vi "action_set.vi"(0 "reference":refnum<class "OSA.lvclass">, 2 "action data":T1[](array[typedef]) {"par 4" format="%.2f"; "par 3" format="%.2f"; "par 2" format="%.2f"; "par" format="%.2f"}, 5 "error in (no error)":errorcluster) -> (14 "duplicate reference":refnum<class "OSA.lvclass">, 19 "error out":errorcluster)   [LabVIEW 2010, in "OSA.lvclass"]
doc: "Set next action and place it in queue."
uses:
  OSA.lvclass
  misc_examples/action_data.ctl
  typeDef/queue_action.ctl
  OSA20X_misc.lvlib
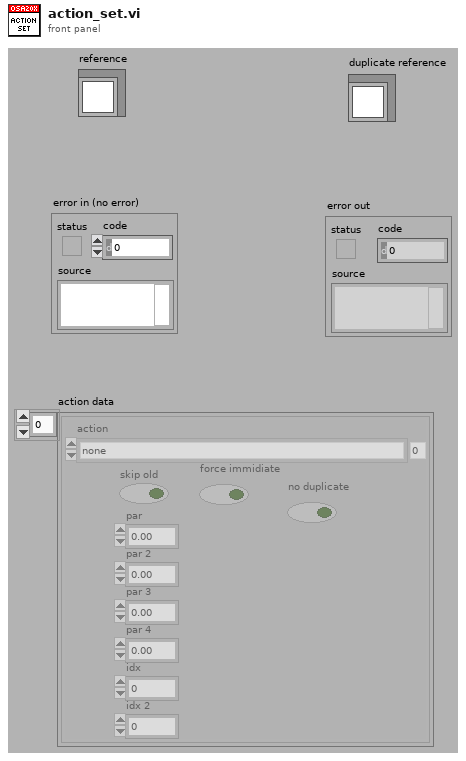
[diagram p1: front panel]
types:
  T1 = typedef "OSA.lvclass/action_data.ctl" = cluster{"action":T2, "skip old":bool, "force immidiate":bool, "par":dbl, "par 2":dbl, "par 3":dbl, "par 4":dbl, "idx":i32, "idx 2":i32, "no duplicate":bool}
  T2 = typedef "OSA.lvclass/queue_action.ctl" = enum16{"none", "stop", "GUI_plotInterferogram", "GUI_plotSpectrum", "GUI_plotInterferogramRescale", "GUI_plotSpectrumRescale", "GUI_plotInterferogramReset", "GUI_plotSpectrumReset", "GUI_plotInterferogramAutoScaleY", "GUI_plotSpectrumAutoScaleY", "GUI_plotInterferogramZoomOut", "GUI_plotSpectrumZoomOut", "GUI_plotInterferogramPane", "GUI_plotSpectrumPane", "GUI_plotInterferogramZoomMouse", "GUI_plotSpectrumZoomMouse", "ENVIRONMENT temperature", "ENVIRONMENT pressure", "MODE_resolution set", "MODE_resolution get", "MODE_sensitivity set", "MODE_sensitivity get", "MODE_PDTemperature set", "MODE_PDTemperature get", "REBOOT/RESET firmware", "ACQASYNC_acquireSingleSpectrum", "ACQASYNC_continuous start", "ACQASYNC_continuous stop\n", "ACQASYNC_get last interferogram", "ACQASYNC_get last spectrum", "ACQASYNC_get last waveNr", "ACQOPT_interferogram smoothing set", "ACQOPT_interferogram smoothing get", "ACQOPT_spectrum smoothing set", "ACQOPT_spectrum smoothing get", "ACQOPT_apodisation type set", "ACQOPT_apodisation type get", "ACQOPT_phase correction type set", "ACQOPT_phase correction type get", "ACQOPT_acqIntervall_set", "ACQOPT_acqIntervall_get", "ACQOPT_average spectrum set", "ACQOPT_average spectrum get", "ACQOPT_rolling average set", "ACQOPT_rolling average get", "ACQOPT_zero fill factor set", "ACQOPT_zero fill factor get", "ACQOPT_cycle counting set", "ACQOPT_cycle counting get", "ACQOPT_air measure option set", "ACQOPT_air measure option get", "ACQOPT_gainLevel auto get", "ACQOPT_gainLevel auto set", "ACQOPT_gainLevel get", "ACQOPT_gainLevel set", "ACQOPT_getAll", "INSTRUMENT_PROPERTY_range_WaveNr_min", "INSTRUMENT_PROPERTY_range_WaveNr_max", "INSTRUMENT_PROPERTY_reference_wavelength_cm^-1", "INSTRUMENT_PROPERTY_samplesPerRefPeriod", "INSTRUMENT_PROPERTY_resolution_waveNrPercm", "INSTRUMENT_PROPERTY_availableGainLevels", "INSTRUMENT_PROPERTY_status", "CONVERT", "ANALYSE_POWER", "ANALYSE_PEAKS", "ANALYSE_WAVELENGTH", "ANALYSE_SPECTRUM", "ANALYSE_INTERFEROGRAM", "ANALYSE_COHERENCE_LENGTH", "MATH", "MATH_power", "MATH_peaks", "FILE", "miscellaneous"}
  T3 = typedef "OSA.lvclass/ObjectAttributes.ctl" = cluster{"Stop":bool, "dataType":T4, "spectrometerIdx":u16, "buffer size interferogram":i32, "interferogram":cluster{"new":bool, "plot_x_ min":sgl, "plot_x_max":sgl, "plot_y_min":sgl, "plot_y_max":sgl, "Graph Intrfrgrm":T5, "timeStamp":u32, "signal (%)":dbl, "traces":cluster{"idx":u32, "broadBand":bool, "monoChromatic":bool, "peakToPeakSignal":dbl, "peakToPeakPos":dbl}[], "traces idx last":i32}, "spectrum":cluster{"new":bool, "plot_x_min":sgl, "plot_x_max":sgl, "plot_unit_x":T6, "plot_unit_y":T7, "plot_y_min":sgl, "plot_y_max":sgl, "Graph Spectrum":T5, "timeStamp":u32, "X_VAL_OPTIONS":enum16{"MIN_MAX", "ARRAY"}, "traces":cluster{"idx":u32}[], "traces idx last":i32}, "Thorlabs_OSA_64.lvclass:queue_action.ctlqueue ref":refnum<queue>, "action":T2, "plot zoom step":dbl, "buffer semaphore":T8, "acq stopped":bool, "dataType active":T4, "temperature (degr C)":sgl, "pressure (hPa)":sgl, "rel humidity (%)":sgl, "settings":cluster{"resolution":T9, "sensitivity":T10, "Average":bool, "average nr":u32, "apodisation":T11, "acq delay (ms)":u32, "airMesure":T12, "wmtr on":bool, "intfgrm_smooth_width":u16, "intfgrm_smooth_nrOfPasses":u16, "intfgrm_smooth":T13, "phaseCorrection":T14, "zeroFill":u8, "spectr_smooth":T13, "spectr_smooth_width":u16, "spectr_smooth_nrOfPasses":u16, "resolution (/cm)":sgl, "REF wavelength, (nm)":dbl, "gain_idx":u16, "gainAuto":bool, "gain_relative":dbl, "PD sensitivity mode":T15, "PD senseMode implemented":bool, "SensorTemperature implemented":bool, "SensorPressure implemented":bool, "SensorHumidity implemented":bool}, "peaks position":sgl[], "peaks width":sgl[], "peaks height":sgl[], "peaks max nr":u32, "peaks latest nr":i32, "peaks new":bool, "power":dbl, "power new":bool, "path":string, "wavelength (WNr)":dbl, "wavelength new":bool, "buffer size spectrum":i32, "status":string, "VI reference":refnum<vi>, "funcPointer":u64, "libraryPointer":u64, "singleAcquisition":bool, "coherenceLength (cm)":dbl, "coherenceLength new":bool, "spectrometer model":string, "spectrometer serial nr":string, "peaks thld left":sgl[], "peaks thld right":sgl[], "coherenceLength error (cm)":dbl, "ADC bits":u16, "peaks position centroid":sgl[], "peaks height centroid":sgl[], "OSA series":T16, "channel index spectrum":u16, "spectrometer rangeLow, (/cm)":dbl, "spectrometer rangeHigh, (/cm)":dbl, "channel index interferogram":u16}
  T4 = typedef "OSA.lvclass/acq_dataType.ctl" = enum16{"none", "interferogram", "spectrum"}
  T5 = typedef "OSA.lvclass/graph_intensity.ctl" = refnum<vi>
  T6 = typedef "OSA.lvclass/spectrum_x_unit.ctl" = enum16{"wavenr/cm", "THz", "eV", "nm_air", "nm_vac"}
  T7 = typedef "OSA.lvclass/y_unit.ctl" = enum16{"ADC counts", "dBm pwr absolute", "dBm pwr density", "mW pwr absolute", "mW pwr density"}
  T8 = typedef "Semaphore RefNum" = refnum<k1>
  T9 = typedef "OSA.lvclass/resolution.ctl" = enum16{"low", "high"}
  T10 = typedef "OSA.lvclass/sensitivityMode.ctl" = enum16{"low", "low medium", "high medium", "high"}
  T11 = typedef "OSA.lvclass/apodisation.ctl" = enum16{"NONE", "NORTON_BEER_WEAK", "NORTON_BEER_MEDIUM", "NORTON_BEER_STRONG", "TRIANGULAR", "COSINE", "HANN", "HAMMING", "BLACKMANHARRIS3", "BLACKMANHARRIS4", "GAUSSIAN"}
  T12 = typedef "OSA.lvclass/airMeasure.ctl" = enum16{"TEMPERATURE", "PRESSURE"}
  T13 = typedef "OSA.lvclass/interferogram_smoothing.ctl" = enum16{"NONE", "BINOMIAL", "SAVITSKY_GOLAY", "FOURIER", "MOVING_AVERAGE", "GAUSSIAN"}
  T14 = typedef "OSA.lvclass/phaseCorrection.ctl" = enum16{"NONE", "MERTZ", "FORMAN", "MERTZ_FILE", "FORMAN_FILE", "FUTURE COMP."}
  T15 = typedef "OSA.lvclass/PDTemperatureMode.ctl" = enum16{"cool: better sensitivity/noise floor", "warm: extended wl range"}
  T16 = typedef "OSA.lvclass/OSA_series.ctl" = enum16{"OSA200", "OSA300", "UNKNOWN"}
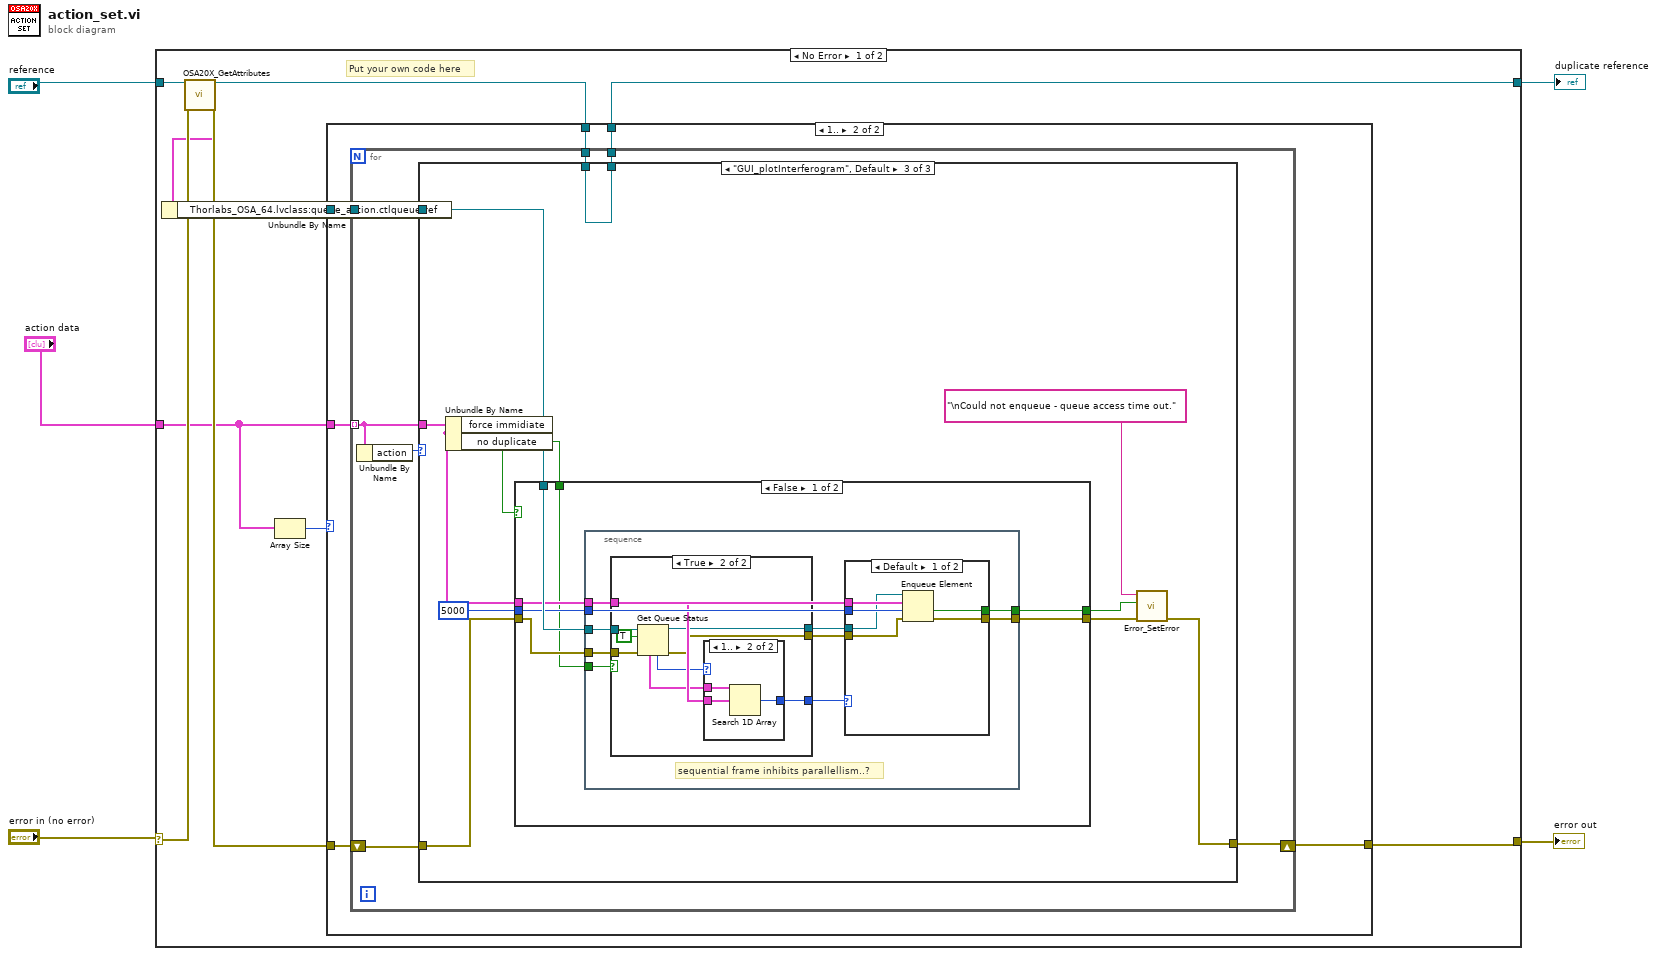
[diagram p0: block diagram]
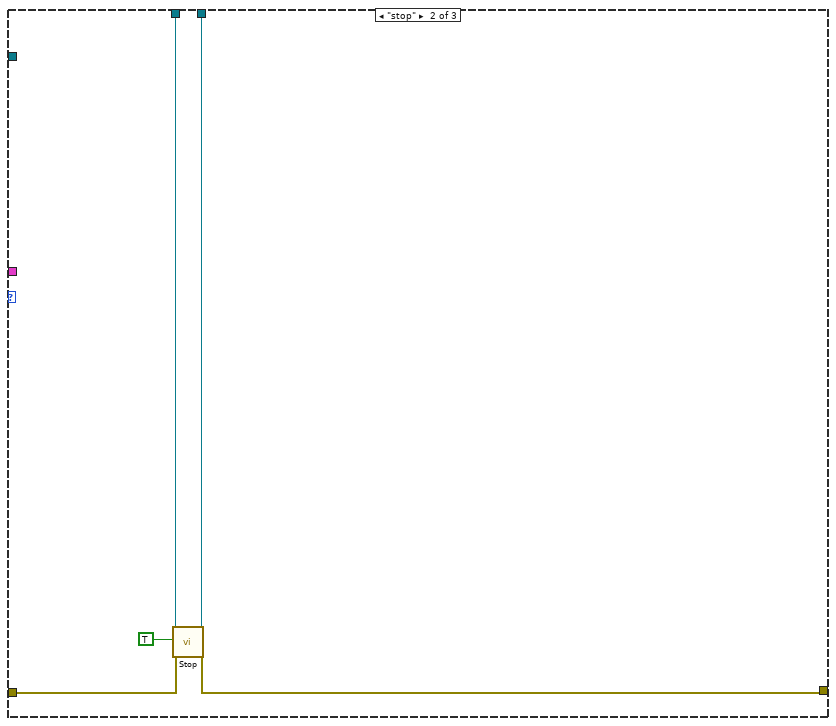
[diagram p4: hidden frame]
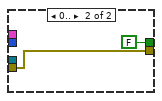
[diagram p5: hidden frame]
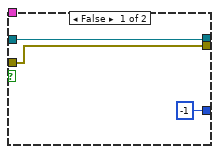
[diagram p6: hidden frame]
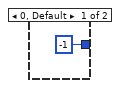
[diagram p7: hidden frame]
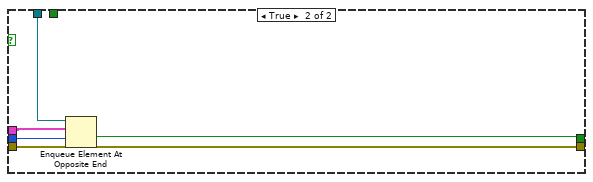
[diagram p8: hidden frame]
diagram:
  n1 = case shown="No Error" "error in (no error)" {
    selector: "error in (no error)" -> [w14 w96]
    tunnel: [w9 w96] -> w5
    tunnel: "reference" -> [w15 w97]
    tunnel: [w10 w97] -> w2
    tunnel: "action data" -> [w8 _]
    frame No Error {
      # "Put your own code here"
      n2 = call "OSA20X_GetAttributes.vi"("reference in"=w15, "error in (no error)"=w14) -> ("reference out"=w11:refnum<class "OSA.lvclass">, "Data"=w6:T3, "error out"=w12:errorcluster)  [unwired: 14 in, 1 out]
      n3 = Unbundle By Name(w6) -> ("Thorlabs_OSA_64.lvclass:queue_action.ctlqueue ref"=w13:refnum<queue>)
      n4 = Array Size(array=w8) -> (size(s)=w7:i32)
      n5 = case shown="1.." w7 {
        tunnel: w13 -> [_ w23]
        tunnel: w12 -> [w16 w19]
        tunnel: w8 -> [_ w22]
        tunnel: w11 -> [w17 w21]
        tunnel: [w17 w20] -> w10
        tunnel: [w16 w18] -> w9
        frame 0, Default {
        }
        frame 1.. {
          n6 = for {
            tunnel: w23 -> [w30]
            tunnel: w22 -> [w24] mode=indexing
            tunnel: w21 -> [w29]
            tunnel: [w28] -> w20
            shift-right: [w27] -> w18
            shift-left: w19 -> [w26]
            n7 = Unbundle By Name(w24) -> ("action"=w25:T2)
            n8 = case shown="\"GUI_plotInterferogram\", Default" w25 {
              tunnel: w30 -> [_ _ w43]
              tunnel: w26 -> [w31 w37 w42]
              tunnel: [w31 w36 w45] -> w27
              tunnel: w24 -> [_ _ w40]
              tunnel: w29 -> [w32 w34 w41]
              tunnel: [w32 w33 w41] -> w28
              frame "none" {
              }
              frame "stop" {
                n9 = call "Stop.vi"("reference"=w34, "Stop"=TRUE, "error in (no error)"=w37) -> ("reference"=w33:refnum<class "OSA.lvclass">, "error out"=w36:errorcluster)  [unwired: 14 in, 1 out]
              }
              frame "GUI_plotInterferogram", Default {
                n10 = Unbundle By Name(w40) -> ("force immidiate"=w39:bool, "no duplicate"=w38:bool)
                n11 = case shown="False" w39 {
                  tunnel: [w55 w94] -> w48
                  tunnel: [w54 w90] -> w47
                  tunnel: 5000 ("timeout in ms (-1)") -> [w51 w93]
                  tunnel: w43 -> [w53 w91]
                  tunnel: w42 -> [w52 w95]
                  tunnel: w40 -> [w50 w92]
                  tunnel: w38 -> [w49 _]
                  frame False {
                    n12 = stacked-sequence {
                      tunnel: [w65] -> w55
                      tunnel: [w64] -> w54
                      tunnel: w53 -> [w63]
                      tunnel: w52 -> [w62]
                      tunnel: w51 -> [w61]
                      tunnel: w50 -> [w60]
                      tunnel: w49 -> [w57]
                      frame #0 {
                        # "sequential frame inhibits parallellism..?"
                        n13 = case shown="True" w57 {
                          tunnel: w63 -> [w75 w85]
                          tunnel: w62 -> [w74 w84]
                          tunnel: w60 -> [_ w83]
                          tunnel: [w75 w80] -> w59
                          tunnel: [w74 w79] -> w58
                          tunnel: [-1 ("index of element") w78] -> w56
                          frame False {
                          }
                          frame True {
                            n14 = Get Queue Status(queue=w85, return elements? (F)=TRUE, error in (no error)=w84) -> (queue out=w80:refnum<queue>, error out=w79:errorcluster, # elements in queue=w82:i32, elements=w81:T1[])  [unwired: 4 out]
                            n15 = case shown="1.." w82 {
                              tunnel: w81 -> [_ w89]
                              tunnel: w83 -> [_ w88]
                              tunnel: [-1 ("index of element") w87] -> w78
                              frame 0, Default {
                              }
                              frame 1.. {
                                n16 = Search 1D Array(1D array=w89, element=w88) -> (index of element=w87:i32)  [unwired: 1 in]
                              }
                            }
                          }
                        }
                        n17 = case shown="Default" w56 {
                          tunnel: [w71 w73] -> w65
                          tunnel: [w70 FALSE ("timed out?")] -> w64
                          tunnel: w61 -> [w69 _]
                          tunnel: w60 -> [w68 _]
                          tunnel: w59 -> [w67 _]
                          tunnel: w58 -> [w66 w73]
                          frame Default {
                            n18 = Enqueue Element(queue=w67, element=w68, timeout in ms (-1)=w69, error in (no error)=w66) -> (timed out?=w70:bool, error out=w71:errorcluster)  [unwired: 1 out]
                          }
                          frame 0.. {
                          }
                        }
                      }
                    }
                  }
                  frame True {
                    n19 = Enqueue Element At Opposite End(queue=w91, element=w92, timeout in ms (-1)=w93, error in (no error)=w95) -> (timed out?=w90:bool, error out=w94:errorcluster)  [unwired: 1 out]
                  }
                }
                n20 = call "Error_SetError.vi"("error in"=w48, "status (true)"=w47, "source(\"\")"="\nCould not enqueue - queue access time out." ("source(\"\")")) -> ("error out"=w45:errorcluster)  [unwired: 4 in]
              }
            }
          }
        }
      }
    }
    frame Error {
      # "Error"
    }
  }
  "error out" <- w5
  "duplicate reference" <- w2
